vi "Set Instance Stop Trigger.vi"(8 "error in (no error)":errorcluster, 9 "Stop Trigger Time":timestamp, 11 "Waveform Log in":refnum<class "Waveform Log.lvclass">) -> (0 "error out":errorcluster, 3 "Waveform Log out":refnum<class "Waveform Log.lvclass">)   [LabVIEW 2015, in "Waveform Data Logger Engine.lvlib" / "Waveform Log.lvclass"]
uses:
  Waveform Log.lvclass
  Waveform Log.lvclass/Waveform Log.ctl
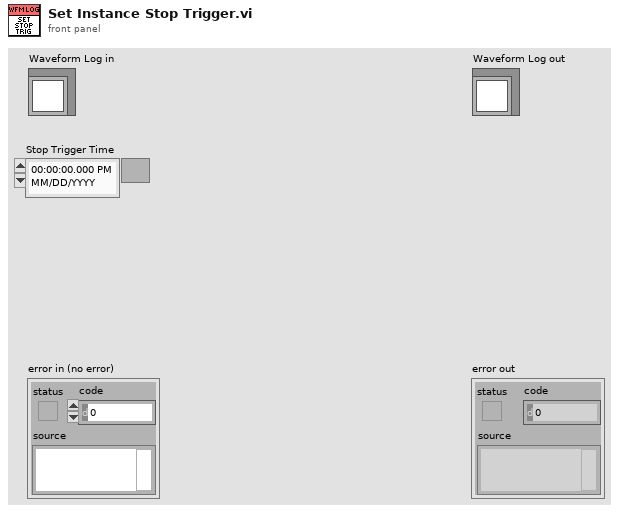
[diagram p1: front panel]
types:
  T1 = typedef "Waveform Data Logger Engine.lvlib/Waveform Log.lvclass/Log Instance.ctl" = cluster{"Segmented Log":refnum<data-value>, "Log Waveforms":T2[], "Log Start":timestamp, "Log Stop":timestamp, "Start Trigger Time":timestamp, "Stop Trigger Time":timestamp, "Time of Last Write":timestamp, "Timeout":dbl, "Stop cmd received":bool}
  T2 = typedef "Waveform Data Logger Engine.lvlib/Waveform Log.lvclass/Log Instance Waveform.ctl" = cluster{"Wfm Info":T3, "Count / Instance":i32, "Previous Segment":u64, "Wfm Complete?":bool, "Last Sample Logged":timestamp, "Data Logged":bool, "Log segmented":bool}
  T3 = typedef "Waveform Data Logger Engine.lvlib/Waveform Log.lvclass/Waveform Information.ctl" = cluster{"Name":string, "Wfm Data Type":T4, "Decimation":u32}
  T4 = typedef "Waveform Data Logger Engine.lvlib/Waveform Log.lvclass/Waveform Data Type.ctl" = enum16{"Double", "ComplexDouble"}
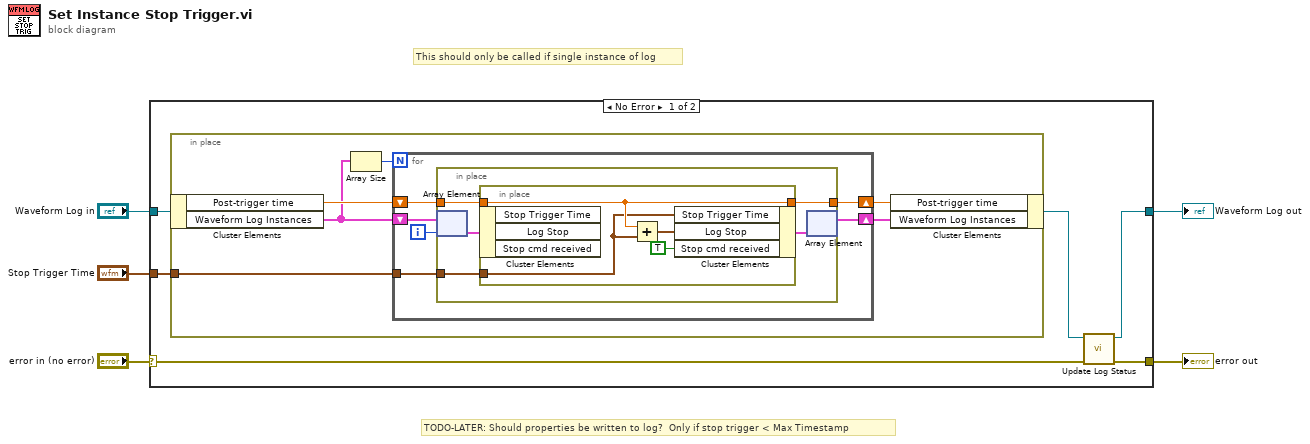
[diagram p0: block diagram]
diagram:
  # "This should only be called if single instance of log"
  # "TODO-LATER: Should properties be written to log?  Only if stop trigger < Max Timestamp"
  n1 = case shown="No Error" "error in (no error)" {
    selector: "error in (no error)" -> [w6 w34]
    tunnel: [w7 w34] -> w4
    tunnel: [w8 w33] -> w2
    tunnel: "Waveform Log in" -> [w11 w33]
    tunnel: "Stop Trigger Time" -> [w10 _]
    frame No Error {
      n2 = in-place {
        in-place-border: w10 -> [w14]
        n3 = in-place-cluster #1(w11) -> ("Post-trigger time"=w16:dbl, "Waveform Log Instances"=w12:T1[])
        n4 = Array Size(array=w12) -> (size(s)=w13:i32)
        n5 = for {
          N: w13 -> [_]
          tunnel: w14 -> [w19]
          shift-right: [w22] -> w17
          shift-left: w12 -> [w23]
          shift-right: [w20] -> w15
          shift-left: w16 -> [w21]
          i -> [w18]
          n6 = in-place {
            in-place-border: w21 -> [w25]
            in-place-border: [w26] -> w20
            in-place-border: w19 -> [w27]
            n7 = in-place-array #2(w23, w18) -> (w28:T1)
            n8 = in-place {
              in-place-border: w27 -> [w30]
              in-place-border: [w32] -> w26
              in-place-border: w25 -> [w32]
              n9 = in-place-cluster #3(w28) -> ()  [unwired: 3 out]
              n10 = Add(x=w32, y=w30) -> (x+y=w31:timestamp)
              n11 = in-place-cluster #3("Stop Trigger Time"=w30, "Log Stop"=w31, "Stop cmd received"=TRUE) -> (w24:T1)
            }
            n12 = in-place-array #2(w24) -> (w22:T1[])  [unwired: 1 out]
          }
        }
        n13 = in-place-cluster #1("Post-trigger time"=w15, "Waveform Log Instances"=w17) -> (w9:refnum<class "Waveform Log.lvclass">)
      }
      n14 = call "Update Log Status.vi"("error in (no error)"=w6, "Waveform Log in"=w9) -> ("error out"=w7:errorcluster, "Waveform Log out"=w8:refnum<class "Waveform Log.lvclass">)  [unwired: 8 in]
    }
    frame Error {
    }
  }
  "error out" <- w4
  "Waveform Log out" <- w2
